vi "Promote Element (U8).vi"(9 "Index to Promote":i32, 11 "Array In":u8[](array[numeric])) -> (3 "Array Out":u8[](array[numeric]))   [LabVIEW 2015, in "ArrayExtensions.lvlib"]
uses:
  ArrayExtensions.lvlib
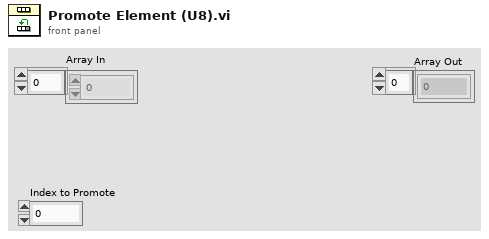
[diagram p1: front panel]
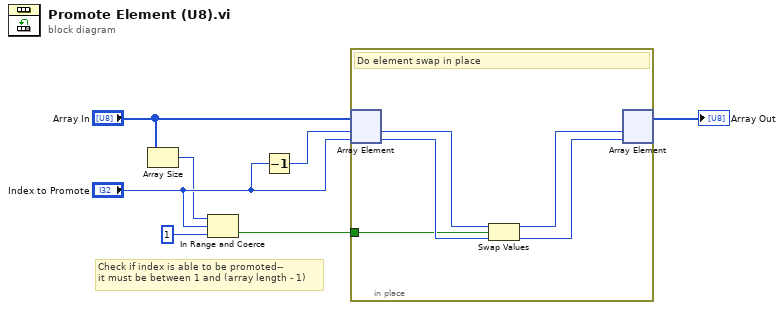
[diagram p0: block diagram]
diagram:
  # "Check if index is able to be promoted--\nit must be between 1 and (array length - 1)"
  n1 = Array Size(array="Array In") -> (size(s)=w2:i32)
  n2 = In Range and Coerce(upper limit=w2, x="Index to Promote", lower limit=1) -> (In Range?=w1:bool)  [unwired: 1 out]
  n3 = Decrement(x="Index to Promote") -> (x-1=w7:i32)
  n4 = in-place {
    in-place-border: w1 -> [w8]
    # "Do element swap in place"
    n5 = in-place-array #1("Array In", w7, "Index to Promote") -> (w12:u8, w11:u8)
    n6 = Swap Values(12:w12, 13:w8, 14:w11) -> (1:w10:u8, 3:w9:u8)
    n7 = in-place-array #1(w10, w9) -> (→"Array Out":u8[])  [unwired: 2 out]
  }
